vi "FGV_Betreibsdaten.vi"(0 "Dynamische Werte":T3, 1 "Sollwert schreiben":T1 {"Ausgangskonzentration\nKomponente 2" format="%#.4f"; "Eingangskonzentration \nKomponente 2" format="%#.4f"; "Ausgangskonzentration \nKomponente 1" format="%#.4f"; "Eingangskonzentration\nKomponente 1" format="%#.4f"; "Eingangskonzentration \nTrägergas" format="%#.4f"; "Gesamtdurchfluss" format="%#.4f"}, 2 "Gase":refnum<vi>, 3 "Sollwerte lesen":T1 {"Ausgangskonzentration\nKomponente 2" format="%#.4f"; "Eingangskonzentration \nKomponente 2" format="%#.4f"; "Ausgangskonzentration \nKomponente 1" format="%#.4f"; "Eingangskonzentration\nKomponente 1" format="%#.4f"; "Eingangskonzentration \nTrägergas" format="%#.4f"; "Gesamtdurchfluss" format="%#.4f"}, 4 "Strings und Werte":cluster{string, i32}[][](array[cluster]), 5 "error in (no error)":errorcluster caption="Fehler (Eingang, kein Fehler)", 6 "Gase schreiben":T2 {"Komponente 2" items=["AI", "BN", "hr", "l"]; "Komponente 1" items=["AR", "SF", "de"]; "Trägergas" items=["AIR", "MG"]}, 8 "Gase lesen":T2 {"Komponente 2" items=["AI", "BN", "hr", "l"]; "Komponente 1" items=["AR", "SF", "de"]; "Trägergas" items=["AIR", "MG"]}, 11 "Enum":T4) -> (10 "Gase schreiben":T2 {"Komponente 2" items=["AI", "BN", "hr", "l"]; "Komponente 1" items=["AR", "SF", "de"]; "Trägergas" items=["AIR", "MG"]}, 12 "Gase lesen":T2 {"Komponente 2" items=["AI", "BN", "hr", "l"]; "Komponente 1" items=["AR", "SF", "de"]; "Trägergas" items=["AIR", "MG"]}, 14 "Dynamische Werte 2":T3, 15 "Sollwerte schreiben":T1 {"Ausgangskonzentration\nKomponente 2" format="%#.4f"; "Eingangskonzentration \nKomponente 2" format="%#.4f"; "Ausgangskonzentration \nKomponente 1" format="%#.4f"; "Eingangskonzentration\nKomponente 1" format="%#.4f"; "Eingangskonzentration \nTrägergas" format="%#.4f"; "Gesamtdurchfluss" format="%#.4f"}, 16 "Array":refnum<vi>[](array[refnum]), 17 "Sollwerte lesen":T1 {"Ausgangskonzentration\nKomponente 2" format="%#.4f"; "Eingangskonzentration \nKomponente 2" format="%#.4f"; "Ausgangskonzentration \nKomponente 1" format="%#.4f"; "Eingangskonzentration\nKomponente 1" format="%#.4f"; "Eingangskonzentration \nTrägergas" format="%#.4f"; "Gesamtdurchfluss" format="%#.4f"}, 18 "Sollwert für Vergleich":T1 {"Ausgangskonzentration\nKomponente 2" format="%#.4f"; "Eingangskonzentration \nKomponente 2" format="%#.4f"; "Ausgangskonzentration \nKomponente 1" format="%#.4f"; "Eingangskonzentration\nKomponente 1" format="%#.4f"; "Eingangskonzentration \nTrägergas" format="%#.4f"; "Gesamtdurchfluss" format="%#.4f"}, 19 "error out":errorcluster caption="Fehler (Ausgang)")   [LabVIEW 2020, in "Linearisierung v2.lvlib" / "Gasteiler.lvlib" / "HovaCal.lvlib"]
uses:
  HovaCal.lvlib
  Dynamsiche_Werte.ctl
  Betriebsdaten.ctl
  Gase.ctl
  Aktion_FGV_Betriebsdaten.ctl
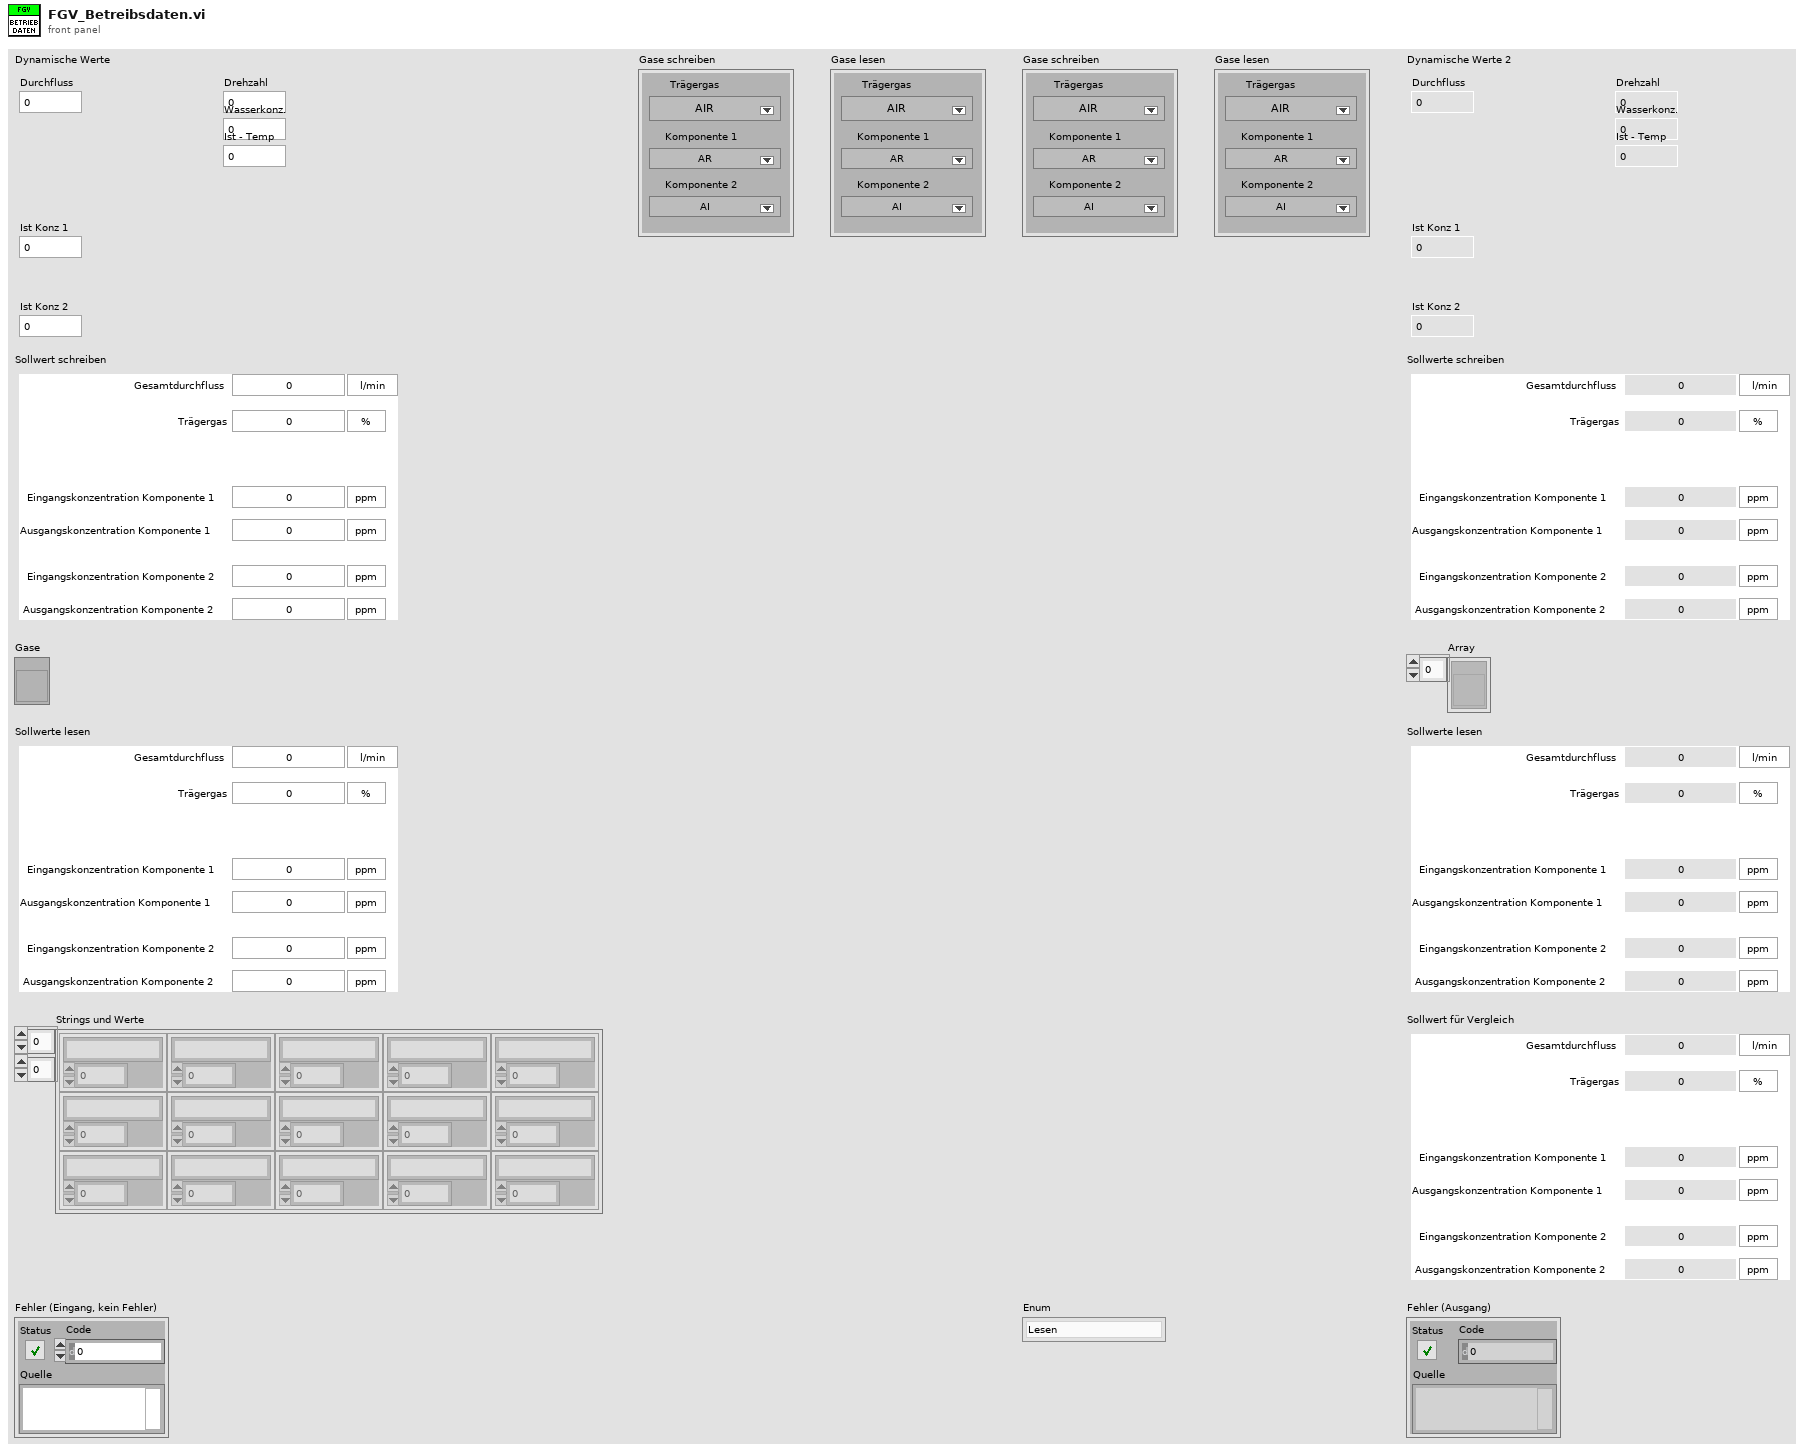
[diagram p1: front panel]
types:
  T1 = typedef "Linearisierung v2.lvlib/Gasteiler.lvlib/HovaCal.lvlib/Betriebsdaten.ctl" = cluster{"Gesamtdurchfluss":dbl, "Eingangskonzentration \nTrägergas":dbl, "Eingangskonzentration\nKomponente 1":dbl, "Eingangskonzentration \nKomponente 2":dbl, "Ausgangskonzentration \nKomponente 1 ":dbl, "Ausgangskonzentration\nKomponente 2":dbl, "l/min -> ml/min":bool, "N2 %->ppm":bool, "Komp1 ppm->%":bool, "Komp2ppm->%":bool, "Sollkomp1ppm->%":bool, "Sollkomp2ppm->%":bool}
  T2 = typedef "Linearisierung v2.lvlib/Gasteiler.lvlib/HovaCal.lvlib/Gase.ctl" = cluster{"Trägergas":u16, "Komponente 1":u16, "Komponente 2":u16}
  T3 = typedef "Linearisierung v2.lvlib/Gasteiler.lvlib/HovaCal.lvlib/Dynamsiche_Werte.ctl" = cluster{"Durchfluss":dbl, "Drehzahl":dbl, "Wasserkonz.":dbl, "Ist - Temp":dbl, "Ist Konz 1":dbl, "Ist Konz 2":dbl}
  T4 = typedef "Linearisierung v2.lvlib/Gasteiler.lvlib/HovaCal.lvlib/Aktion_FGV_Betriebsdaten.ctl" = enum16{"Lesen", "Sollwerte schreiben", "Sollwerte lesen", "Gase schreiben", "Gase lesen", "Dynamische Werte", "GaseRef", "Gase aendern"}
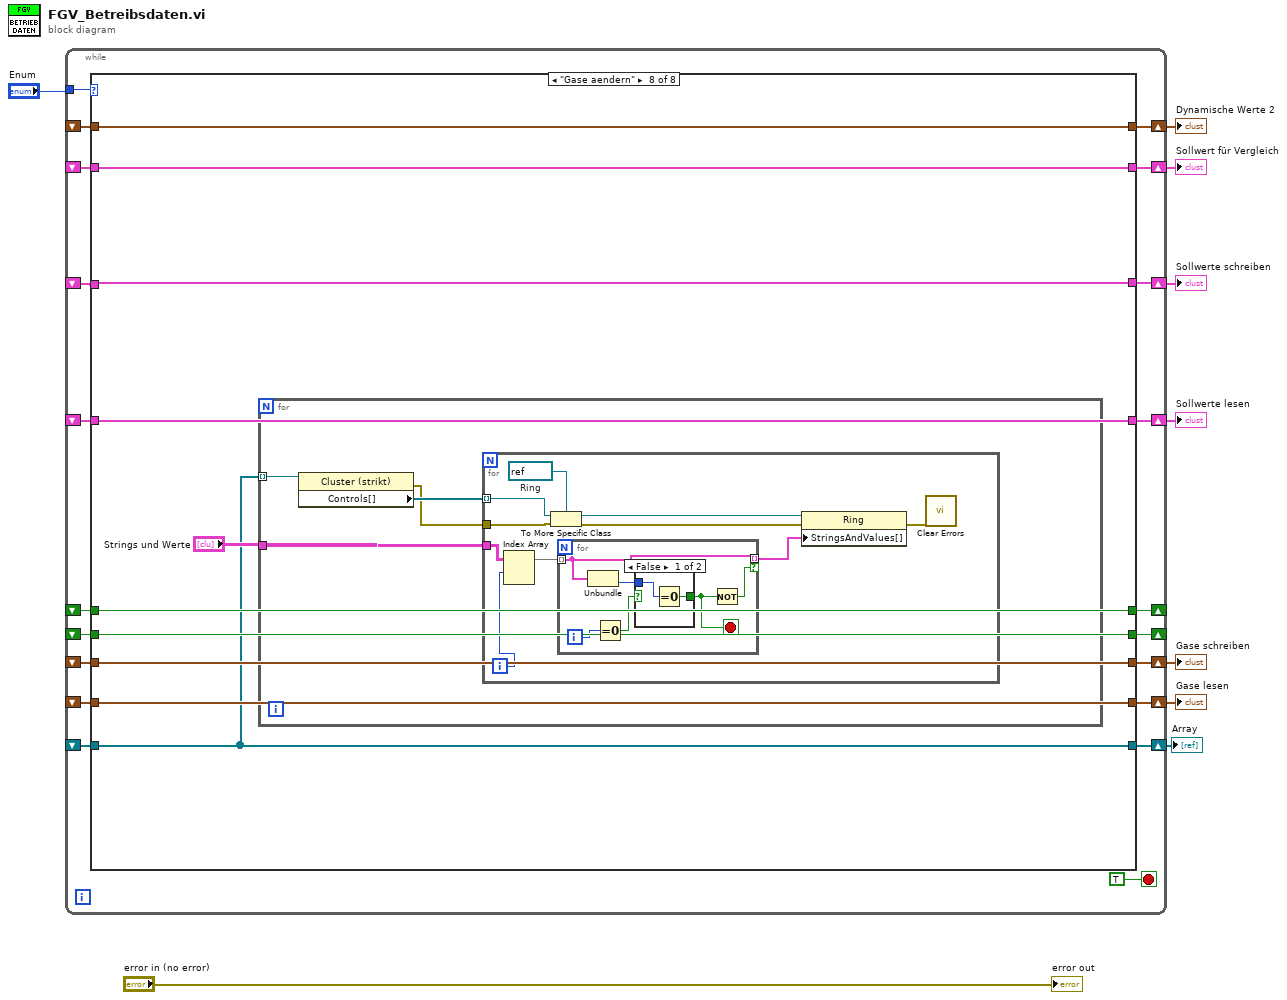
[diagram p0: block diagram]
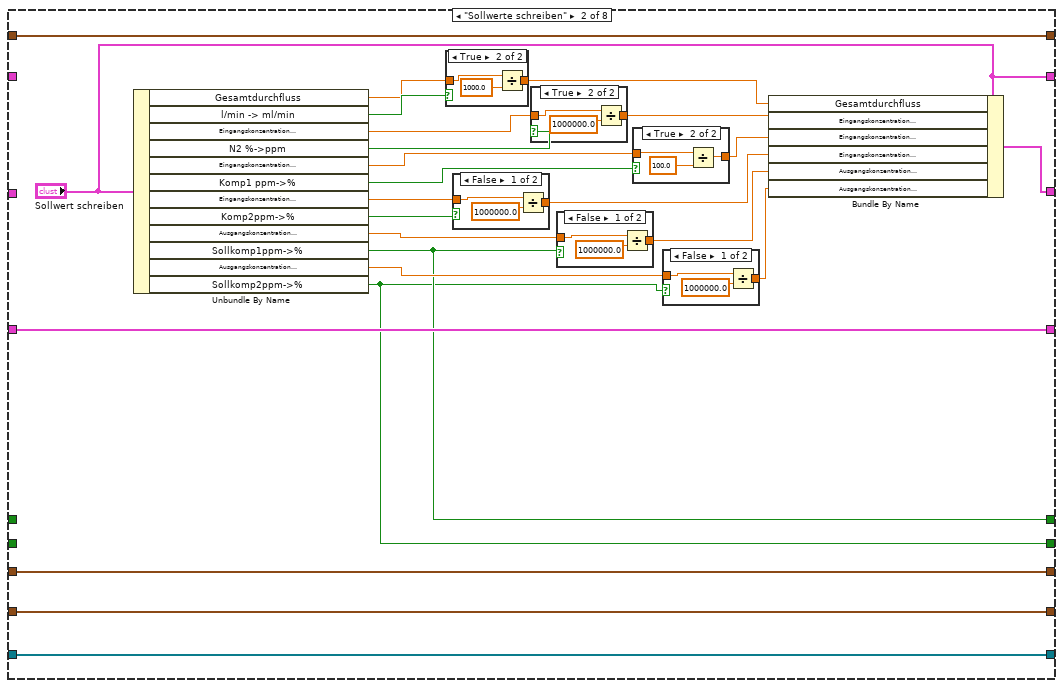
[diagram p3: hidden frame]
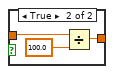
[diagram p4: hidden frame]
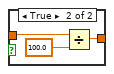
[diagram p5: hidden frame]
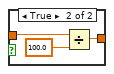
[diagram p6: hidden frame]
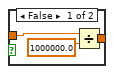
[diagram p7: hidden frame]
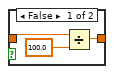
[diagram p8: hidden frame]
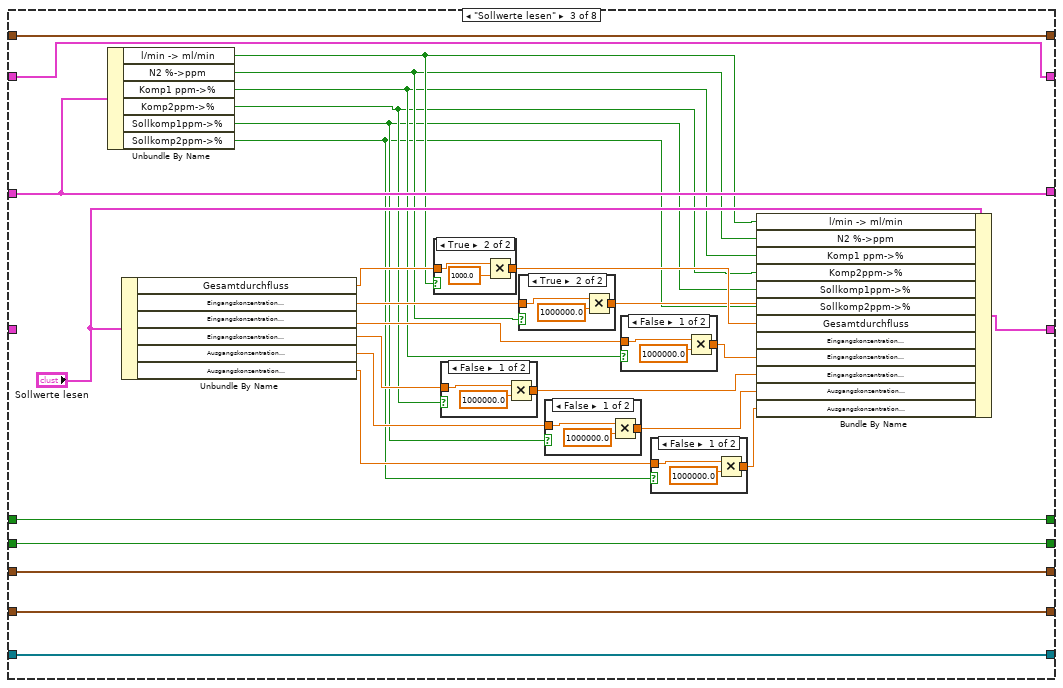
[diagram p10: hidden frame]
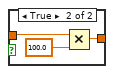
[diagram p11: hidden frame]
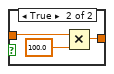
[diagram p12: hidden frame]
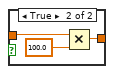
[diagram p13: hidden frame]
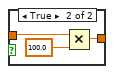
[diagram p14: hidden frame]
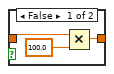
[diagram p15: hidden frame]
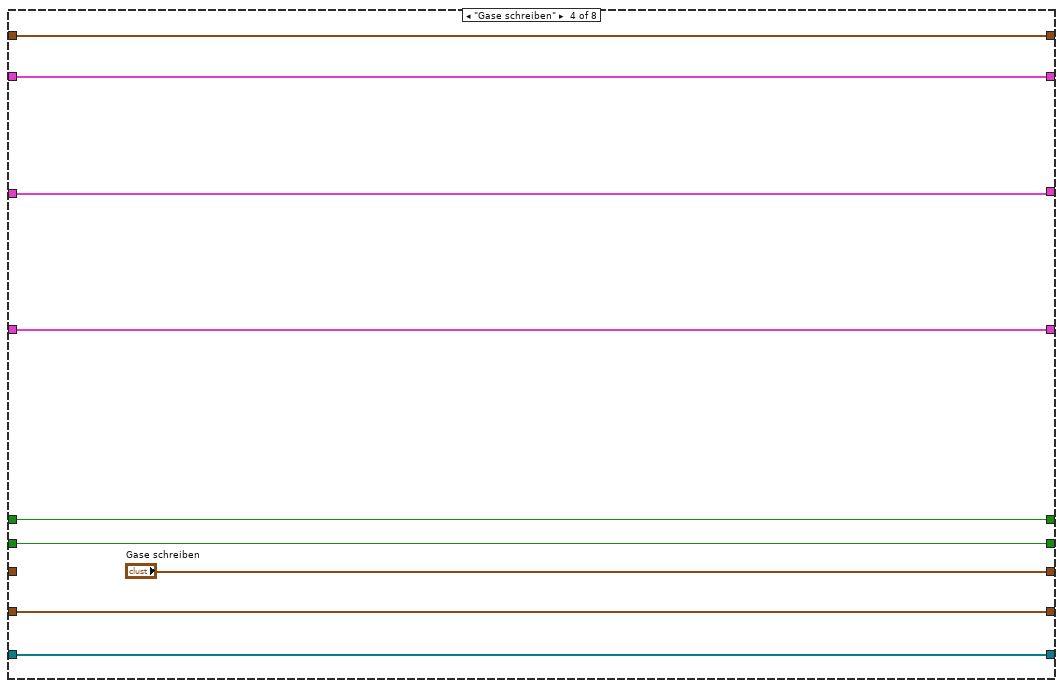
[diagram p17: hidden frame]
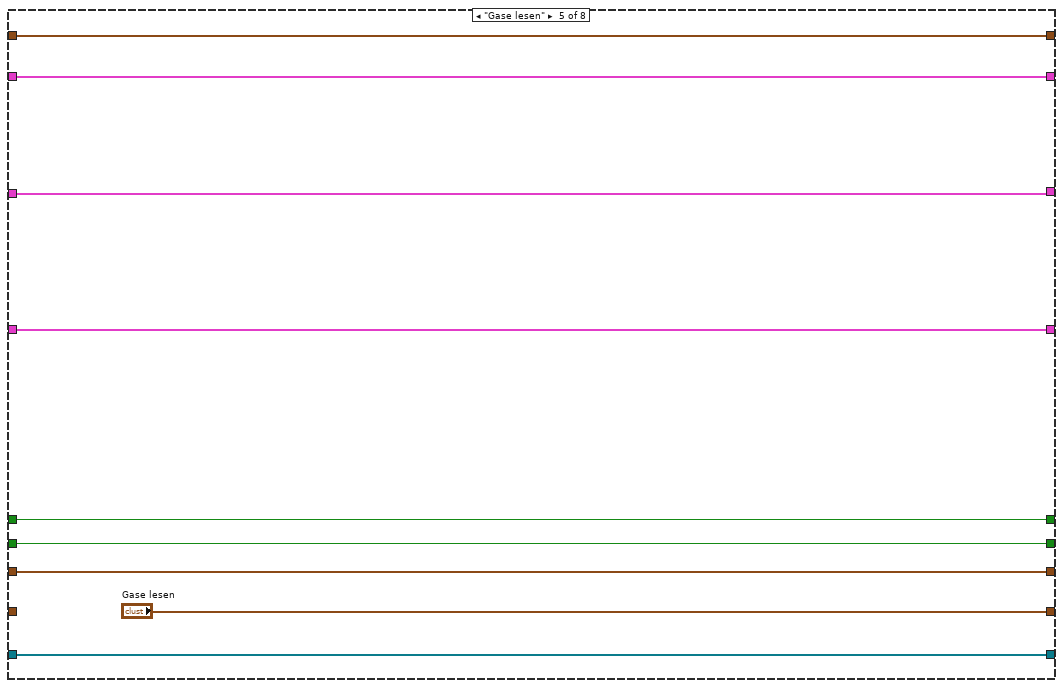
[diagram p18: hidden frame]
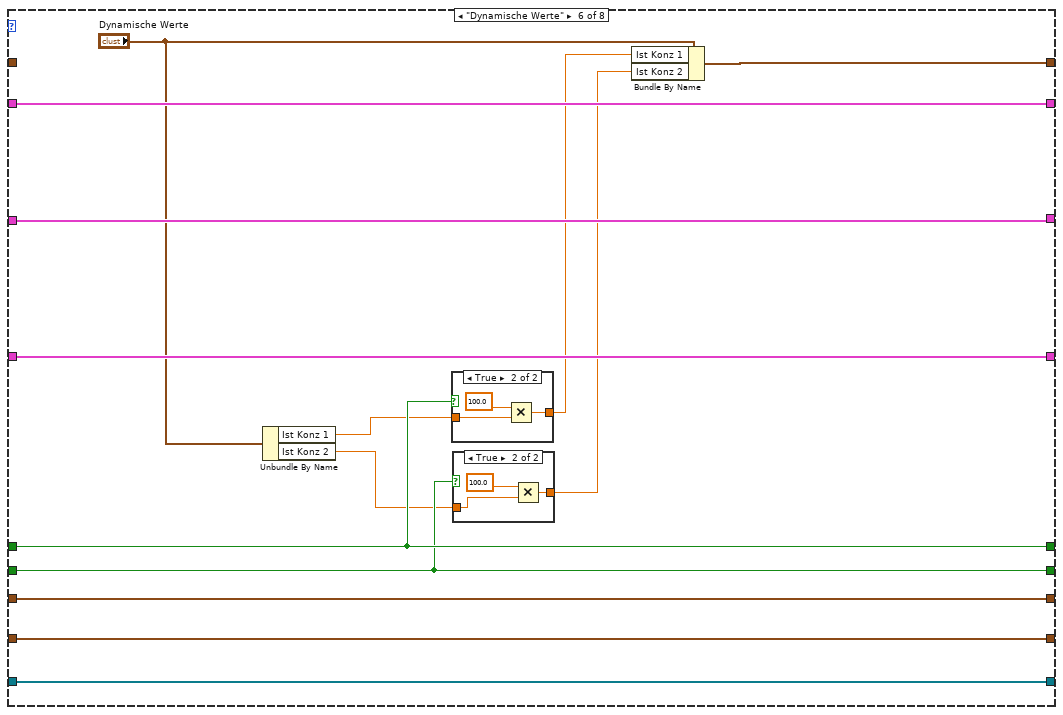
[diagram p19: hidden frame]
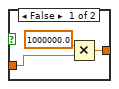
[diagram p20: hidden frame]
diagram:
  n1 = while {
    shift-right: [w28] -> w8
    shift-left: _ -> [w23]
    shift-right: [w27] -> w7
    shift-left: _ -> [w22]
    shift-right: [w26] -> w6
    shift-left: _ -> [w21]
    shift-right: [w25] -> w5
    shift-left: _ -> [w20]
    shift-right: [w24] -> w3
    shift-left: _ -> [w19]
    tunnel: "Enum" -> [w18]
    shift-right: [w17] -> w2
    shift-left: _ -> [w16]
    shift-right: [w15] -> _
    shift-left: _ -> [w13]
    shift-right: [w14] -> _
    shift-left: _ -> [w12]
    shift-right: [w11] -> w1
    shift-left: _ -> [w10]
    stop <- TRUE stop-if-true
    n2 = case shown="\"Gase aendern\"" w18 {
      tunnel: [w38 w63 w125 w167 w176 w179 w207 w225] -> w28
      tunnel: [w37 w44 w120 w166 w175 w191 w209 w223] -> w27
      tunnel: [w36 w62 w121 w165 w174 w190 w210 w222] -> w26
      tunnel: [w35 w61 w124 "Gase schreiben" w173 w189 w212 w221] -> w25
      tunnel: [w34 w60 w123 w164 "Gase lesen" w188 w211 w220] -> w24
      tunnel: w23 -> [w38 w63 w125 w167 w176 _ w207 w225]
      tunnel: w22 -> [w37 _ w120 w166 w175 w191 w209 w223]
      tunnel: w21 -> [w36 w62 _ w165 w174 w190 w210 w222]
      tunnel: w20 -> [w35 w61 w124 _ w173 w189 w212 w221]
      tunnel: w19 -> [w34 w60 w123 w164 _ w188 w211 w220]
      tunnel: [w33 "Sollwert schreiben" w107 w163 w172 w187 w208 w224] -> w17
      tunnel: w16 -> [w33 _ w107 w163 w172 w187 w208 w224]
      tunnel: [w32 w41 w100 w162 w171 w186 w217 w227] -> w15
      tunnel: [w31 w40 w99 w161 w170 w184 w216 w226] -> w14
      tunnel: w13 -> [w32 _ w100 w162 w171 w186 w217 w227]
      tunnel: w12 -> [w31 _ w99 w161 w170 w184 w216 w226]
      tunnel: [w30 w39 w98 w160 w169 w178 w206 w218] -> w11
      tunnel: w10 -> [w30 w39 w98 w160 w169 w178 _ w218]
      frame "Lesen", Default {
      }
      frame "Sollwerte schreiben" {
        n3 = Unbundle By Name("Sollwert schreiben") -> ("Gesamtdurchfluss"=w58:dbl, "l/min -> ml/min"=w59:bool, "Eingangskonzentration \nTrägergas"=w55:dbl, "N2 %->ppm"=w56:bool, "Eingangskonzentration\nKomponente 1"=w53:dbl, "Komp1 ppm->%"=w42:bool, "Eingangskonzentration \nKomponente 2"=w52:dbl, "Komp2ppm->%"=w51:bool, "Ausgangskonzentration \nKomponente 1"=w50:dbl, "Sollkomp1ppm->%"=w41:bool, "Ausgangskonzentration\nKomponente 2"=w49:dbl, "Sollkomp2ppm->%"=w40:bool)
        n4 = case shown="True" w59 {
          tunnel: w58 -> [w94 w96]
          tunnel: [w94 w97] -> w57
          frame False {
          }
          frame True {
            n5 = Divide(x=w96, y=sgl 1000.0) -> (x/y=w97:dbl)
          }
        }
        n6 = case shown="False" w51 {
          tunnel: w52 -> [w76 w79]
          tunnel: [w78 w80] -> w47
          frame False {
            n7 = Divide(x=w76, y=sgl 1000000.0) -> (x/y=w78:dbl)
          }
          frame True {
            n8 = Divide(x=w79, y=sgl 100.0) -> (x/y=w80:dbl)
          }
        }
        n9 = case shown="True" w56 {
          tunnel: w55 -> [w88 w91]
          tunnel: [w89 w93] -> w54
          frame False {
            n10 = Divide(x=w88, y=sgl 100.0) -> (x/y=w89:dbl)
          }
          frame True {
            n11 = Divide(x=w91, y=sgl 1000000.0) -> (x/y=w93:dbl)
          }
        }
        n12 = case shown="False" w41 {
          tunnel: w50 -> [w70 w73]
          tunnel: [w72 w74] -> w46
          frame False {
            n13 = Divide(x=w70, y=sgl 1000000.0) -> (x/y=w72:dbl)
          }
          frame True {
            n14 = Divide(x=w73, y=sgl 100.0) -> (x/y=w74:dbl)
          }
        }
        n15 = case shown="True" w42 {
          tunnel: w53 -> [w82 w85]
          tunnel: [w84 w86] -> w48
          frame False {
            n16 = Divide(x=w82, y=sgl 1000000.0) -> (x/y=w84:dbl)
          }
          frame True {
            n17 = Divide(x=w85, y=sgl 100.0) -> (x/y=w86:dbl)
          }
        }
        n18 = case shown="False" w40 {
          tunnel: w49 -> [w64 w67]
          tunnel: [w66 w68] -> w45
          frame False {
            n19 = Divide(x=w64, y=sgl 1000000.0) -> (x/y=w66:dbl)
          }
          frame True {
            n20 = Divide(x=w67, y=sgl 100.0) -> (x/y=w68:dbl)
          }
        }
        n21 = Bundle By Name(cluster="Sollwert schreiben", "Gesamtdurchfluss"=w57, "Eingangskonzentration \nTrägergas"=w54, "Eingangskonzentration\nKomponente 1"=w48, "Eingangskonzentration \nKomponente 2"=w47, "Ausgangskonzentration \nKomponente 1"=w46, "Ausgangskonzentration\nKomponente 2"=w45) -> (w44:T1)
      }
      frame "Sollwerte lesen" {
        n22 = Unbundle By Name(w120) -> ("l/min -> ml/min"=w106:bool, "N2 %->ppm"=w105:bool, "Komp1 ppm->%"=w104:bool, "Komp2ppm->%"=w103:bool, "Sollkomp1ppm->%"=w102:bool, "Sollkomp2ppm->%"=w101:bool)
        n23 = Unbundle By Name("Sollwerte lesen") -> ("Gesamtdurchfluss"=w119:dbl, "Eingangskonzentration \nTrägergas"=w117:dbl, "Eingangskonzentration\nKomponente 1"=w115:dbl, "Eingangskonzentration \nKomponente 2"=w114:dbl, "Ausgangskonzentration \nKomponente 1"=w113:dbl, "Ausgangskonzentration\nKomponente 2"=w112:dbl)
        n24 = case shown="True" w106 {
          tunnel: w119 -> [w156 w158]
          tunnel: [w156 w159] -> w118
          frame False {
          }
          frame True {
            n25 = Multiply(x=w158, y=sgl 1000.0) -> (x*y=w159:dbl)
          }
        }
        n26 = case shown="False" w103 {
          tunnel: w114 -> [w138 w141]
          tunnel: [w140 w142] -> w110
          frame False {
            n27 = Multiply(x=w138, y=sgl 1000000.0) -> (x*y=w140:dbl)
          }
          frame True {
            n28 = Multiply(x=w141, y=sgl 100.0) -> (x*y=w142:dbl)
          }
        }
        n29 = case shown="True" w105 {
          tunnel: w117 -> [w150 w153]
          tunnel: [w151 w155] -> w116
          frame False {
            n30 = Multiply(x=w150, y=sgl 100.0) -> (x*y=w151:dbl)
          }
          frame True {
            n31 = Multiply(x=w153, y=sgl 1000000.0) -> (x*y=w155:dbl)
          }
        }
        n32 = case shown="False" w102 {
          tunnel: w113 -> [w132 w135]
          tunnel: [w134 w136] -> w109
          frame False {
            n33 = Multiply(x=w132, y=sgl 1000000.0) -> (x*y=w134:dbl)
          }
          frame True {
            n34 = Multiply(x=w135, y=sgl 100.0) -> (x*y=w136:dbl)
          }
        }
        n35 = case shown="False" w104 {
          tunnel: w115 -> [w144 w147]
          tunnel: [w146 w148] -> w111
          frame False {
            n36 = Multiply(x=w144, y=sgl 1000000.0) -> (x*y=w146:dbl)
          }
          frame True {
            n37 = Multiply(x=w147, y=sgl 100.0) -> (x*y=w148:dbl)
          }
        }
        n38 = case shown="False" w101 {
          tunnel: w112 -> [w126 w129]
          tunnel: [w128 w130] -> w108
          frame False {
            n39 = Multiply(x=w126, y=sgl 1000000.0) -> (x*y=w128:dbl)
          }
          frame True {
            n40 = Multiply(x=w129, y=sgl 100.0) -> (x*y=w130:dbl)
          }
        }
        n41 = Bundle By Name(cluster="Sollwerte lesen", "l/min -> ml/min"=w106, "N2 %->ppm"=w105, "Komp1 ppm->%"=w104, "Komp2ppm->%"=w103, "Sollkomp1ppm->%"=w102, "Sollkomp2ppm->%"=w101, "Gesamtdurchfluss"=w118, "Eingangskonzentration \nTrägergas"=w116, "Eingangskonzentration\nKomponente 1"=w111, "Eingangskonzentration \nKomponente 2"=w110, "Ausgangskonzentration \nKomponente 1"=w109, "Ausgangskonzentration\nKomponente 2"=w108) -> (w121:T1)
      }
      frame "Gase schreiben" {
      }
      frame "Gase lesen" {
      }
      frame "Dynamische Werte" {
        n42 = Unbundle By Name("Dynamische Werte") -> ("Ist Konz 1"=w185:dbl, "Ist Konz 2"=w183:dbl)
        n43 = case shown="True" w186 {
          tunnel: w185 -> [w199 w201]
          tunnel: [w198 w203] -> w181
          frame False {
            n44 = Multiply(x=sgl 1000000.0, y=w199) -> (x*y=w198:dbl)
          }
          frame True {
            n45 = Multiply(x=sgl 100.0, y=w201) -> (x*y=w203:dbl)
          }
        }
        n46 = case shown="True" w184 {
          tunnel: w183 -> [w193 w195]
          tunnel: [w192 w196] -> w180
          frame False {
            n47 = Multiply(x=sgl 1000000.0, y=w193) -> (x*y=w192:dbl)
          }
          frame True {
            n48 = Multiply(x=sgl 100.0, y=w195) -> (x*y=w196:dbl)
          }
        }
        n49 = Bundle By Name(cluster="Dynamische Werte", "Ist Konz 1"=w181, "Ist Konz 2"=w180) -> (w179:T3)
      }
      frame "GaseRef" {
        n50 = control-ref of="Gase schreiben"() -> (w215:refnum<vi>)
        n51 = control-ref of="Gase lesen"() -> (w214:refnum<vi>)
        n52 = control-ref of="Gase schreiben"() -> (w205:refnum<vi>)
        n53 = control-ref of="Gase lesen"() -> (w204:refnum<vi>)
        n54 = Build Array(w215, w214, "Gase", w205, w204) -> (w206:refnum<vi>[])
      }
      frame "Gase aendern" {
        n55 = for {
          tunnel: w218 -> [w231] mode=indexing
          tunnel: "Strings und Werte" -> [w228]
          n56 = property class="Cluster (strikt)"(reference=w231) -> (error out=w229:errorcluster, "Controls[]"=w230:refnum<vi>[])  [unwired: 1 in, 1 out]
          n57 = for {
            tunnel: w230 -> [w237] mode=indexing
            tunnel: w229 -> [w236]
            tunnel: w228 -> [w235]
            i -> [w232]
            w239 = refnum<vi> refnum  # Ring
            n58 = Index Array(array=w235, index (row)=w232) -> (element=w233:cluster{string, i32}[])  [unwired: 1 in]
            n59 = To More Specific Class(target class=w239, reference=w237, error in=w236) -> (specific class reference=w240:refnum<vi>, error out=w241:errorcluster)
            n60 = for {
              tunnel: w233 -> [w244] mode=indexing
              tunnel: [w244] -> w234 mode=indexing if=w242
              i -> [w247]
              stop <- w243 stop-if-true
              n61 = Unbundle(w244) -> (w245:i32)  [unwired: 1 out]
              n62 = Equal To 0?(x=w247) -> (x = 0?=w246:bool)
              n63 = case shown="False" w246 {
                tunnel: w245 -> [w249 _]
                tunnel: [w248 FALSE] -> w243
                frame False {
                  n64 = Equal To 0?(x=w249) -> (x = 0?=w248:bool)
                }
                frame True {
                }
              }
              n65 = Not(x=w243) -> (.not. x?=w242:bool)
            }
            n66 = property class="Ring"(reference=w240, error in=w241, "StringsAndValues[]"=w234) -> (error out=w238:errorcluster)  [unwired: 1 out]
            n67 = call <vilib>:"Clear Errors.vi"("error in (no error)"=w238) -> ()  [unwired: 5 in, 2 out]
          }
        }
      }
    }
  }
  "Dynamische Werte 2" <- w8
  "Sollwerte schreiben" <- w7
  "Sollwerte lesen" <- w6
  "Gase schreiben" <- w5
  "Gase lesen" <- w3
  "Sollwert für Vergleich" <- w2
  "Array" <- w1
  "error out" <- "error in (no error)"
